vi "PH_IEEE1394Camera.open Cam.vi"(0 "VI in":refnum<vi>, 5 "error in (no error)":errorcluster) -> (14 "VI out":refnum<vi>, 16 "Cam Session Out":T1, 18 "Cam Error out":errorcluster, 19 "error out":errorcluster)   [LabVIEW 2014, in "PH_IEEE1394Camera.lvlib"]
uses:
  PH_IEEE1394Camera.lvlib
  <vilib>/userdefined/High Color/IMAQdx.ctl
  <vilib>/vision/driver/NI_Vision_Acquisition_Software.lvlib
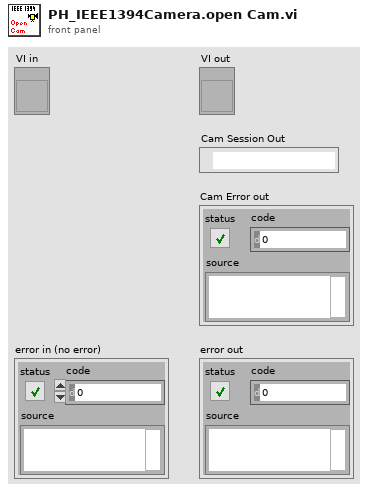
[diagram p1: front panel]
types:
  T1 = typedef "IMAQdx.ctl" = refnum<k21>
  T2 = typedef "PH_IEEE1394Camera.lvlib/PH_IEEE1394Camera.i attribute.ctl" = cluster{"Gui Refs":cluster{"Brightness":refnum<vi>, "Shutter":refnum<vi>, "Gain":refnum<vi>, "Center of Gravity":refnum<vi>, "Supported Video Modes":refnum<vi>, "Trigger Polarity":refnum<vi>, "Trigger Mode":refnum<vi>, "Trigger Timeout":refnum<vi>, "Bit Depth":refnum<vi>, "Video Mode":refnum<vi>, "Top":refnum<vi>, "Bottom":refnum<vi>, "Left":refnum<vi>, "Right":refnum<vi>, "Set ROI to Maximum":refnum<vi>, "Camera Details":refnum<vi>, "Current Cam Attributes":refnum<vi>, "Attribute to set":refnum<vi>, "Num Value":refnum<vi>, "String Value":refnum<vi>, "Bool Value":refnum<vi>, "Set Cam Attribute":refnum<vi>}, "Cam":cluster{"IMAQ1394 Session":T1, "Camera Details":T3}, "Current Attributes":T4[], "Supported Video Modes ":cluster{"Video Mode":u32, "Video Mode Name":string}[], "Wanted Attributes":cluster{"Name":string, "Num Value":dbl, "String Value":string, "Boolean Value":bool}[], "Cam Attributes":T6}
  T3 = typedef "PH_IEEE1394Camera.lvlib/PH_IEEE1394Camera.Cam Details.ctl" = cluster{"Model":string, "Serial Number":dbl, "Cam name (Machinery)":string, "Bus Type":string}
  T4 = typedef "PH_IEEE1394Camera.lvlib/PH_IEEE1394Camera.Cam Attribute.ctl" = cluster{"Information":cluster{"Type":T5, "Readable":bool, "Writable":bool, "Name":string}, "Num Value":dbl, "String Value":string, "Maximum":dbl, "Minimum":dbl, "Units":string, "Description":string, "EnumStrings[]":string[], "EnumValues[]":u32[], "Boolean Value":bool}
  T5 = typedef "NI_Vision_Acquisition_Software.lvlib/IMAQdx Attribute Type.ctl" = enum32{"U32", "I64", "DBL", "String", "Enum", "Bool", "Command"}
  T6 = typedef "PH_IEEE1394Camera.lvlib/PH_IEEE1394Camera.Relevant Cam Attributes.ctl" = cluster{"Video Mode":cluster{"Name":string, "Index":i32}, "Brightness":cluster{"Name":string, "Index":i32}, "Gain":cluster{"Name":string, "Index":i32}, "Shutter":cluster{"Name":string, "Index":i32}, "Trigger Pol":cluster{"Name":string, "Index":i32}, "Trigger Mode":cluster{"Name":string, "Index":i32}, "Timeout":cluster{"Name":string, "Index":i32}, "Bit Depth":cluster{"Name":string, "Index":i32}, "Pixel Bits":cluster{"Name":string, "Index":i32}, "Pixel Bytes":cluster{"Name":string, "Index":i32}, "Left":cluster{"Name":string, "Index":i32}, "Right":cluster{"Name":string, "Index":i32}, "Top":cluster{"Name":string, "Index":i32}, "Bottom":cluster{"Name":string, "Index":i32}}
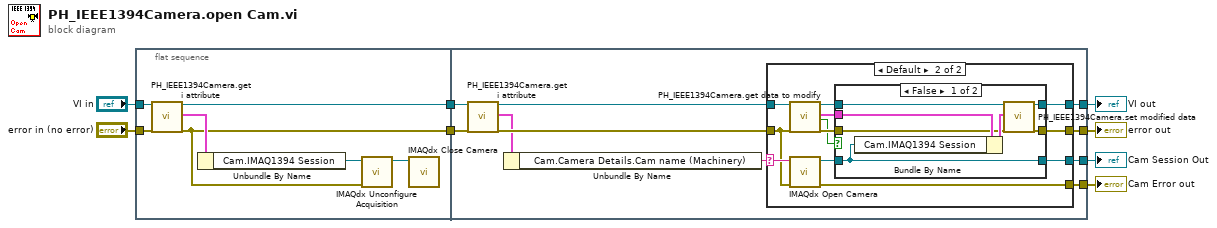
[diagram p0: block diagram]
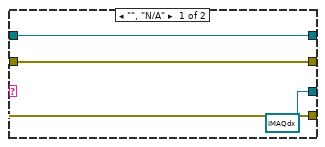
[diagram p2: hidden frame]
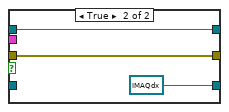
[diagram p3: hidden frame]
diagram:
  n1 = flat-sequence {
    tunnel: [w12] -> w4
    tunnel: "VI in" -> [w11]
    tunnel: "error in (no error)" -> [w10]
    tunnel: [w9] -> w1
    tunnel: [w24] -> w8
    tunnel: [w23] -> w7
    tunnel: [w21] -> w6
    tunnel: [w20] -> w5
    tunnel: w4 -> [w17]
    tunnel: w1 -> [w16]
    frame #0 {
      n2 = call "PH_IEEE1394Camera.get i attribute.vi"("i ref in"=w11, "error in (no error)"=w10) -> ("i ref out"=w12:refnum<vi>, "i attribute"=w14:T2, "error out"=w9:errorcluster)  [unwired: 15 in]
      n3 = Unbundle By Name(w14) -> ("Cam.IMAQ1394 Session"=w15:T1)
      n4 = call <vilib>:"IMAQdx Unconfigure Acquisition.vi"("error in"=w9, "Session In"=w15) -> ("Session Out"=w13:T1)  [unwired: 8 in, 1 out]
      n5 = call <vilib>:"IMAQdx Close Camera.vi"("Session In"=w13) -> ()  [unwired: 10 in, 1 out]
    }
    frame #1 {
      n6 = call "PH_IEEE1394Camera.get i attribute.vi"("i ref in"=w17, "error in (no error)"=w16) -> ("i ref out"=w22:refnum<vi>, "i attribute"=w18:T2, "error out"=w19:errorcluster)  [unwired: 15 in]
      n7 = Unbundle By Name(w18) -> ("Cam.Camera Details.Cam name (Machinery)"=w25:string)
      n8 = case shown="Default" w25 {
        selector: w25 -> [_ w31]
        tunnel: w19 -> [w27 w29]
        tunnel: [T1 refnum ("Session Out") w30] -> w20
        tunnel: [w27 w39] -> w21
        tunnel: w22 -> [w28 w34]
        tunnel: [w28 w33] -> w23
        tunnel: [w27 w32] -> w24
        frame "", "N/A" {
        }
        frame Default {
          n9 = call "PH_IEEE1394Camera.get data to modify.vi"("i ref in"=w34, "error in (no error)"=w29) -> ("i ref out"=w35:refnum<vi>, "i attribute"=w36:T2, "timed out"=w37:bool, "error out"=w38:errorcluster)  [unwired: 14 in]
          n10 = call <vilib>:"IMAQdx Open Camera.vi"("error in"=w29, "Session In"=w31) -> ("error out"=w39:errorcluster, "Session Out"=w40:T1)  [unwired: 8 in]
          n11 = case shown="False" w37 {
            tunnel: w38 -> [w42 w49]
            tunnel: w35 -> [w47 w50]
            tunnel: [w46 w50] -> w33
            tunnel: [w45 w49] -> w32
            tunnel: w36 -> [w43 _]
            tunnel: w40 -> [w41 _]
            tunnel: [w41 T1 refnum ("Session Out")] -> w30
            frame False {
              n12 = Bundle By Name(cluster=w43, "Cam.IMAQ1394 Session"=w41) -> (w44:T2)
              n13 = call "PH_IEEE1394Camera.set modified data.vi"("i ref in"=w47, "i attribute"=w44, "error in (no error)"=w42) -> ("i ref out"=w46:refnum<vi>, "error out"=w45:errorcluster)  [unwired: 15 in]
            }
            frame True {
            }
          }
        }
      }
    }
  }
  "error out" <- w8
  "VI out" <- w7
  "Cam Error out" <- w6
  "Cam Session Out" <- w5
